vi "SIM_FrameProperties.vi"(10 "file path (dialog if empty)":path) -> (0 "data":dbl[][](array[numeric]), 1 "Surf Loc (m)":dbl, 2 "Frame Properties (m)":T1)   [LabVIEW 2021]
uses:
  <vilib>/Utility/file.llb/Read Delimited Spreadsheet (DBL).vi
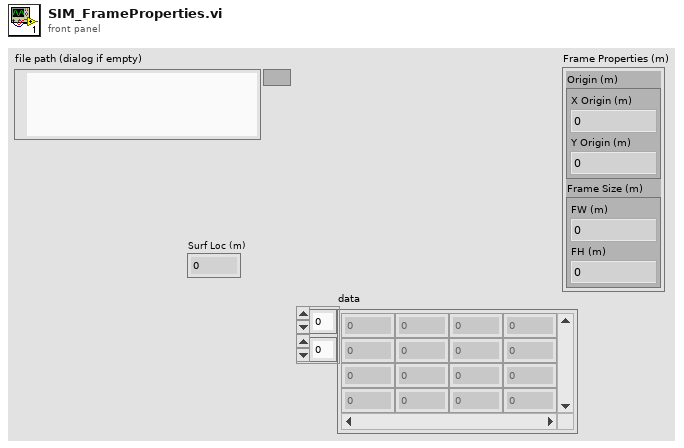
[diagram p1: front panel]
types:
  T1 = cluster{"Origin (m)":cluster{"X Origin (m)":dbl, "Y Origin (m)":dbl}, "Frame Size (m)":cluster{"FW (m)":dbl, "FH (m)":dbl}}
  T2 = cluster{"[0]":dbl, "[1]":dbl, "[2]":dbl, "[3]":dbl, "[4]":dbl, "[5]":dbl, "[6]":dbl, "[7]":dbl, "[8]":dbl}
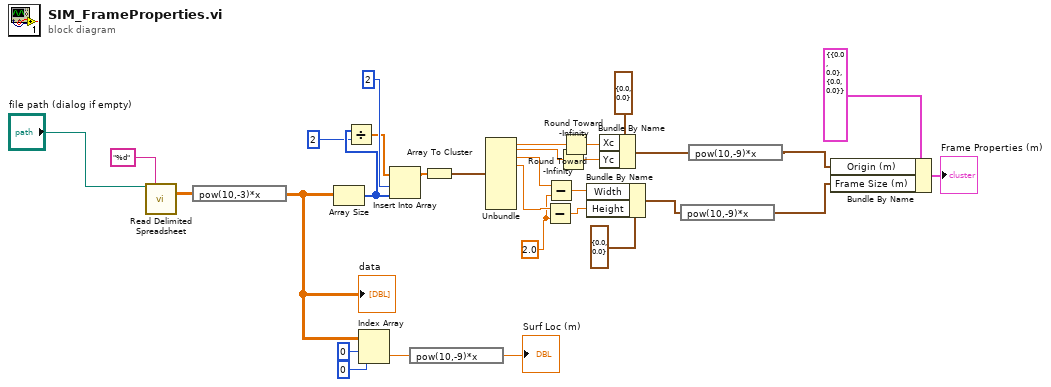
[diagram p0: block diagram]
diagram:
  w5 = 2.0 ("y")
  n1 = call-poly <vilib>:"Read Delimited Spreadsheet.vi"("file path (dialog if empty)"="file path (dialog if empty)", "format (%.3f)"="%d") -> ("all rows"=w26:dbl[][])  [unwired: 8 in, 5 out]
  n2 = expression code="pow(10,-3)*x"(w26) -> (w25:dbl[][])
  "data" <- w25
  n3 = Array Size(array=w25) -> (size(s)=w19:i32[])
  n4 = Divide(x=w19, y=2) -> (x/y=w20:dbl[])
  n5 = Index Array(array=w25, index (row)=0, index (col)=0 ("disabled index (col)")) -> (element=w23:dbl)
  n6 = Insert Into Array(array=w20, index=2, new element=w19) -> (w30:dbl[])
  n7 = expression code="pow(10,-9)*x"(w23) -> (→"Surf Loc (m)":dbl)
  n8 = Array To Cluster(array=w30) -> (cluster=w29:T2)
  n9 = Unbundle(w29) -> ("[0]"=w4:dbl, "[1]"=w1:dbl, "[2]"=w8:dbl, "[3]"=w6:dbl)  [unwired: 5 out]
  n10 = Subtract(x=w6, y=w5) -> (x-y=w7:dbl)
  n11 = Subtract(x=w8, y=w5) -> (x-y=w9:dbl)
  n12 = Round Toward -Infinity(1:w1) -> (0:w2:dbl)
  n13 = Round Toward -Infinity(1:w4) -> (0:w3:dbl)
  n14 = Bundle By Name(cluster=cluster{"Width":sgl, "Height":sgl} {"Width"=0.0, "Height"=0.0} ("Size (m)"), "Width"=w9, "Height"=w7) -> (w16:cluster{"Width":sgl, "Height":sgl})
  n15 = Bundle By Name(cluster=cluster{"Xc":sgl, "Yc":sgl} {"Xc"=0.0, "Yc"=0.0} ("Center coordinates (m)"), "Xc"=w3, "Yc"=w2) -> (w22:cluster{"Xc":sgl, "Yc":sgl})
  n16 = expression code="pow(10,-9)*x"(w16) -> (w12:cluster{"Width":sgl, "Height":sgl})
  n17 = expression code="pow(10,-9)*x"(w22) -> (w13:cluster{"Xc":sgl, "Yc":sgl})
  n18 = Bundle By Name(cluster=T1 {"Origin (m)"={"X Origin (m)"=0.0, "Y Origin (m)"=0.0}, "Frame Size (m)"={"FW (m)"=0.0, "FH (m)"=0.0}} ("Frame Properties (m)"), "Origin (m)"=w13, "Frame Size (m)"=w12) -> (→"Frame Properties (m)":T1)
